vi "Mod_OFDM_Read_Configuration_From_File.vi"(0 "Configuration in":variant, 11 "error in":errorcluster) -> (4 "Configuration out":variant=variant("C"=variant(cluster{"Sub Carrier Selection":cluster{"Sub Carrier":bool, "Data Source":u16, "Modulator":u16}[], "OFDM Parameters":cluster{"# of Sub Carrier":i32, "Length Of Cylic Prefix":i32}} {"Sub Carrier Selection"=[{"Sub Carrier"=TRUE, "Data Source"=0, "Modulator"=0}, {"Sub Carrier"=TRUE, "Data Source"=0, "Modulator"=0}, {"Sub Carrier"=TRUE, "Data Source"=0, "Modulator"=0}, {"Sub Carrier"=TRUE, "Data Source"=0, "Modulator"=0}, {"Sub Carrier"=TRUE, "Data Source"=0, "Modulator"=0}, {"Sub Carrier"=TRUE, "Data Source"=0, "Modulator"=0}, {"Sub Carrier"=TRUE, "Data Source"=0, "Modulator"=0}, {"Sub Carrier"=TRUE, "Data Source"=0, "Modulator"=0}, {"Sub Carrier"=TRUE, "Data Source"=0, "Modulator"=0}, {"Sub Carrier"=TRUE, "Data Source"=0, "Modulator"=0}, {"Sub Carrier"=FALSE, "Data Source"=0, "Modulator"=0}, {"Sub Carrier"=FALSE, "Data Source"=0, "Modulator"=0}, {"Sub Carrier"=FALSE, "Data Source"=0, "Modulator"=0}, {"Sub Carrier"=FALSE, "Data Source"=0, "Modulator"=0}, {"Sub Carrier"=FALSE, "Data Source"=0, "Modulator"=0}, {"Sub Carrier"=FALSE, "Data Source"=0, "Modulator"=0}, {"Sub Carrier"=FALSE, "Data Source"=0, "Modulator"=0}, {"Sub Carrier"=FALSE, "Data Source"=0, "Modulator"=0}, {"Sub Carrier"=FALSE, "Data Source"=0, "Modulator"=0}, {"Sub Carrier"=FALSE, "Data Source"=0, "Modulator"=0}, {"Sub Carrier"=FALSE, "Data Source"=0, "Modulator"=0}, {"Sub Carrier"=FALSE, "Data Source"=0, "Modulator"=0}, {"Sub Carrier"=FALSE, "Data Source"=0, "Modulator"=0}, {"Sub Carrier"=FALSE, "Data Source"=0, "Modulator"=0}, {"Sub Carrier"=FALSE, "Data Source"=0, "Modulator"=0}, {"Sub Carrier"=FALSE, "Data Source"=0, "Modulator"=0}, {"Sub Carrier"=FALSE, "Data Source"=0, "Modulator"=0}, {"Sub Carrier"=FALSE, "Data Source"=0, "Modulator"=0}, {"Sub Carrier"=FALSE, "Data Source"=0, "Modulator"=0}, {"Sub Carrier"=FALSE, "Data Source"=0, "Modulator"=0}, {"Sub Carrier"=FALSE, "Data Source"=0, "Modulator"=0}, {"Sub Carrier"=TRUE, "Data Source"=0, "Modulator"=0}, {"Sub Carrier"=TRUE, "Data Source"=0, "Modulator"=0}, {"Sub Carrier"=TRUE, "Data Source"=0, "Modulator"=0}, {"Sub Carrier"=TRUE, "Data Source"=0, "Modulator"=0}, {"Sub Carrier"=TRUE, "Data Source"=0, "Modulator"=0}, {"Sub Carrier"=TRUE, "Data Source"=0, "Modulator"=0}, {"Sub Carrier"=TRUE, "Data Source"=0, "Modulator"=0}, {"Sub Carrier"=TRUE, "Data Source"=0, "Modulator"=0}, {"Sub Carrier"=TRUE, "Data Source"=0, "Modulator"=0}, {"Sub Carrier"=TRUE, "Data Source"=0, "Modulator"=0}, {"Sub Carrier"=TRUE, "Data Source"=0, "Modulator"=0}, {"Sub Carrier"=TRUE, "Data Source"=0, "Modulator"=0}, {"Sub Carrier"=TRUE, "Data Source"=0, "Modulator"=0}, {"Sub Carrier"=TRUE, "Data Source"=0, "Modulator"=0}, {"Sub Carrier"=TRUE, "Data Source"=0, "Modulator"=0}, {"Sub Carrier"=TRUE, "Data Source"=0, "Modulator"=0}, {"Sub Carrier"=TRUE, "Data Source"=0, "Modulator"=0}, {"Sub Carrier"=TRUE, "Data Source"=0, "Modulator"=0}, {"Sub Carrier"=TRUE, "Data Source"=0, "Modulator"=0}, {"Sub Carrier"=TRUE, "Data Source"=0, "Modulator"=0}, {"Sub Carrier"=TRUE, "Data Source"=0, "Modulator"=0}, {"Sub Carrier"=TRUE, "Data Source"=0, "Modulator"=0}, {"Sub Carrier"=TRUE, "Data Source"=0, "Modulator"=0}, {"Sub Carrier"=TRUE, "Data Source"=0, "Modulator"=0}, {"Sub Carrier"=TRUE, "Data Source"=0, "Modulator"=0}, {"Sub Carrier"=TRUE, "Data Source"=0, "Modulator"=0}, {"Sub Carrier"=TRUE, "Data Source"=0, "Modulator"=0}, {"Sub Carrier"=TRUE, "Data Source"=0, "Modulator"=0}, {"Sub Carrier"=TRUE, "Data Source"=0, "Modulator"=0}, {"Sub Carrier"=TRUE, "Data Source"=0, "Modulator"=0}, {"Sub Carrier"=TRUE, "Data Source"=0, "Modulator"=0}, {"Sub Carrier"=TRUE, "Data Source"=0, "Modulator"=0}, {"Sub Carrier"=TRUE, "Data Source"=0, "Modulator"=0}], "OFDM Parameters"={"# of Sub Carrier"=64, "Length Of Cylic Prefix"=16}}), "Data Source Pool "=variant(cluster{"mode (PN)":enum16{"PN", "pattern", "user"}, "PN sequence order (9)":i32, "base bit pattern (00001111)":enum16{"0", "1", "01", "0011", "00001111"}, "User base bit pattern":i8[]}[] [{"mode (PN)"=enum."PN", "PN sequence order (9)"=9, "base bit pattern (00001111)"=enum."00001111", "User base bit pattern"=[]}, {"mode (PN)"=enum."PN", "PN sequence order (9)"=9, "base bit pattern (00001111)"=enum."00001111", "User base bit pattern"=[]}, {"mode (PN)"=enum."PN", "PN sequence order (9)"=9, "base bit pattern (00001111)"=enum."00001111", "User base bit pattern"=[]}, {"mode (PN)"=enum."PN", "PN sequence order (9)"=9, "base bit pattern (00001111)"=enum."00001111", "User base bit pattern"=[]}, {"mode (PN)"=enum."PN", "PN sequence order (9)"=9, "base bit pattern (00001111)"=enum."00001111", "User base bit pattern"=[]}, {"mode (PN)"=enum."PN", "PN sequence order (9)"=9, "base bit pattern (00001111)"=enum."00001111", "User base bit pattern"=[]}]), "FRAME Table"=variant(string[][] [["C", "1"]]), "Modulator Source Pool "=variant(cluster{"M-QAM":enum16{"4", "16", "64", "256", "1024"}, "M-PSK":enum16{"2", "4", "8", "16", "32", "64", "128", "256"}, "Type of Modulation":enum16{"PSK", "QAM"}, "PSK":cluster{"differential PSK":enum16{"disable", "enable"}, "PSK type":u16}}[] [{"M-QAM"=enum."4", "M-PSK"=enum."4", "Type of Modulation"=enum."PSK", "PSK"={"differential PSK"=enum."disable", "PSK type"=0}}, {"M-QAM"=enum."4", "M-PSK"=enum."4", "Type of Modulation"=enum."PSK", "PSK"={"differential PSK"=enum."disable", "PSK type"=0}}, {"M-QAM"=enum."4", "M-PSK"=enum."4", "Type of Modulation"=enum."PSK", "PSK"={"differential PSK"=enum."disable", "PSK type"=0}}, {"M-QAM"=enum."4", "M-PSK"=enum."4", "Type of Modulation"=enum."PSK", "PSK"={"differential PSK"=enum."disable", "PSK type"=0}}, {"M-QAM"=enum."4", "M-PSK"=enum."4", "Type of Modulation"=enum."PSK", "PSK"={"differential PSK"=enum."disable", "PSK type"=0}}, {"M-QAM"=enum."4", "M-PSK"=enum."2", "Type of Modulation"=enum."PSK", "PSK"={"differential PSK"=enum."disable", "PSK type"=0}}]), "OFDM Frame"=variant(cluster{"Symbol Name":string, "# of Symbols":i32}[] [{"Symbol Name"="C", "# of Symbols"=1}]), "OFDM SYMBOL POOL"=variant(string[] ["C"]), "Pulse Shaping"=variant(cluster{"System Filter":cluster{"TX Filter":enum16{"none", "Raised Cosine", "Root Raised Cos"}, "Alpha":dbl, "filter length":i32}, "Modulation system parameters":cluster{"samples per symbol (16)":i32}, "symbol rate (Hz)":dbl} {"System Filter"={"TX Filter"=enum."Raised Cosine", "Alpha"=0.5, "filter length"=8}, "Modulation system parameters"={"samples per symbol (16)"=16}, "symbol rate (Hz)"=1.0}), "Sub Carrier Selection"=variant(cluster{"Sub Carrier Selection":cluster{"Sub Carrier":bool, "Data Source":u16, "Modulator":u16}[], "OFDM Parameters":cluster{"# of Sub Carrier":i32, "Length Of Cylic Prefix":i32}} {"Sub Carrier Selection"=[{"Sub Carrier"=TRUE, "Data Source"=0, "Modulator"=0}, {"Sub Carrier"=TRUE, "Data Source"=0, "Modulator"=0}, {"Sub Carrier"=TRUE, "Data Source"=0, "Modulator"=0}, {"Sub Carrier"=TRUE, "Data Source"=0, "Modulator"=0}, {"Sub Carrier"=TRUE, "Data Source"=0, "Modulator"=0}, {"Sub Carrier"=TRUE, "Data Source"=0, "Modulator"=0}, {"Sub Carrier"=TRUE, "Data Source"=0, "Modulator"=0}, {"Sub Carrier"=TRUE, "Data Source"=0, "Modulator"=0}, {"Sub Carrier"=TRUE, "Data Source"=0, "Modulator"=0}, {"Sub Carrier"=TRUE, "Data Source"=0, "Modulator"=0}, {"Sub Carrier"=TRUE, "Data Source"=0, "Modulator"=0}, {"Sub Carrier"=TRUE, "Data Source"=0, "Modulator"=0}, {"Sub Carrier"=TRUE, "Data Source"=0, "Modulator"=0}, {"Sub Carrier"=TRUE, "Data Source"=0, "Modulator"=0}, {"Sub Carrier"=TRUE, "Data Source"=0, "Modulator"=0}, {"Sub Carrier"=TRUE, "Data Source"=0, "Modulator"=0}, {"Sub Carrier"=TRUE, "Data Source"=0, "Modulator"=0}, {"Sub Carrier"=TRUE, "Data Source"=0, "Modulator"=0}, {"Sub Carrier"=TRUE, "Data Source"=0, "Modulator"=0}, {"Sub Carrier"=TRUE, "Data Source"=0, "Modulator"=0}, {"Sub Carrier"=TRUE, "Data Source"=0, "Modulator"=0}, {"Sub Carrier"=TRUE, "Data Source"=0, "Modulator"=0}, {"Sub Carrier"=TRUE, "Data Source"=0, "Modulator"=0}, {"Sub Carrier"=TRUE, "Data Source"=0, "Modulator"=0}, {"Sub Carrier"=TRUE, "Data Source"=0, "Modulator"=0}, {"Sub Carrier"=TRUE, "Data Source"=0, "Modulator"=0}, {"Sub Carrier"=TRUE, "Data Source"=0, "Modulator"=0}, {"Sub Carrier"=TRUE, "Data Source"=0, "Modulator"=0}, {"Sub Carrier"=TRUE, "Data Source"=0, "Modulator"=0}, {"Sub Carrier"=TRUE, "Data Source"=0, "Modulator"=0}, {"Sub Carrier"=TRUE, "Data Source"=0, "Modulator"=0}, {"Sub Carrier"=TRUE, "Data Source"=0, "Modulator"=0}, {"Sub Carrier"=TRUE, "Data Source"=0, "Modulator"=0}, {"Sub Carrier"=TRUE, "Data Source"=0, "Modulator"=0}, {"Sub Carrier"=TRUE, "Data Source"=0, "Modulator"=0}, {"Sub Carrier"=TRUE, "Data Source"=0, "Modulator"=0}, {"Sub Carrier"=TRUE, "Data Source"=0, "Modulator"=0}, {"Sub Carrier"=TRUE, "Data Source"=0, "Modulator"=0}, {"Sub Carrier"=TRUE, "Data Source"=0, "Modulator"=0}, {"Sub Carrier"=TRUE, "Data Source"=0, "Modulator"=0}, {"Sub Carrier"=TRUE, "Data Source"=0, "Modulator"=0}, {"Sub Carrier"=TRUE, "Data Source"=0, "Modulator"=0}, {"Sub Carrier"=TRUE, "Data Source"=0, "Modulator"=0}, {"Sub Carrier"=TRUE, "Data Source"=0, "Modulator"=0}, {"Sub Carrier"=TRUE, "Data Source"=0, "Modulator"=0}, {"Sub Carrier"=TRUE, "Data Source"=0, "Modulator"=0}, {"Sub Carrier"=TRUE, "Data Source"=0, "Modulator"=0}, {"Sub Carrier"=TRUE, "Data Source"=0, "Modulator"=0}, {"Sub Carrier"=TRUE, "Data Source"=0, "Modulator"=0}, {"Sub Carrier"=TRUE, "Data Source"=0, "Modulator"=0}, {"Sub Carrier"=TRUE, "Data Source"=0, "Modulator"=0}, {"Sub Carrier"=TRUE, "Data Source"=0, "Modulator"=0}, {"Sub Carrier"=TRUE, "Data Source"=0, "Modulator"=0}, {"Sub Carrier"=TRUE, "Data Source"=0, "Modulator"=0}, {"Sub Carrier"=TRUE, "Data Source"=0, "Modulator"=0}, {"Sub Carrier"=TRUE, "Data Source"=0, "Modulator"=0}, {"Sub Carrier"=TRUE, "Data Source"=0, "Modulator"=0}, {"Sub Carrier"=TRUE, "Data Source"=0, "Modulator"=0}, {"Sub Carrier"=TRUE, "Data Source"=0, "Modulator"=0}, {"Sub Carrier"=TRUE, "Data Source"=0, "Modulator"=0}, {"Sub Carrier"=TRUE, "Data Source"=0, "Modulator"=0}, {"Sub Carrier"=TRUE, "Data Source"=0, "Modulator"=0}, {"Sub Carrier"=TRUE, "Data Source"=0, "Modulator"=0}, {"Sub Carrier"=TRUE, "Data Source"=0, "Modulator"=0}, {"Sub Carrier"=TRUE, "Data Source"=0, "Modulator"=0}, {"Sub Carrier"=TRUE, "Data Source"=0, "Modulator"=0}, {"Sub Carrier"=TRUE, "Data Source"=0, "Modulator"=0}, {"Sub Carrier"=TRUE, "Data Source"=0, "Modulator"=0}, {"Sub Carrier"=TRUE, "Data Source"=0, "Modulator"=0}, {"Sub Carrier"=TRUE, "Data Source"=0, "Modulator"=0}, {"Sub Carrier"=TRUE, "Data Source"=0, "Modulator"=0}, {"Sub Carrier"=TRUE, "Data Source"=0, "Modulator"=0}, {"Sub Carrier"=TRUE, "Data Source"=0, "Modulator"=0}, {"Sub Carrier"=TRUE, "Data Source"=0, "Modulator"=0}, {"Sub Carrier"=TRUE, "Data Source"=0, "Modulator"=0}, {"Sub Carrier"=TRUE, "Data Source"=0, "Modulator"=0}, {"Sub Carrier"=TRUE, "Data Source"=0, "Modulator"=0}, {"Sub Carrier"=TRUE, "Data Source"=0, "Modulator"=0}, {"Sub Carrier"=TRUE, "Data Source"=0, "Modulator"=0}, {"Sub Carrier"=TRUE, "Data Source"=0, "Modulator"=0}, {"Sub Carrier"=TRUE, "Data Source"=0, "Modulator"=0}, {"Sub Carrier"=TRUE, "Data Source"=0, "Modulator"=0}, {"Sub Carrier"=TRUE, "Data Source"=0, "Modulator"=0}, {"Sub Carrier"=TRUE, "Data Source"=0, "Modulator"=0}, {"Sub Carrier"=TRUE, "Data Source"=0, "Modulator"=0}, {"Sub Carrier"=TRUE, "Data Source"=0, "Modulator"=0}, {"Sub Carrier"=TRUE, "Data Source"=0, "Modulator"=0}, {"Sub Carrier"=TRUE, "Data Source"=0, "Modulator"=0}, {"Sub Carrier"=TRUE, "Data Source"=0, "Modulator"=0}, {"Sub Carrier"=TRUE, "Data Source"=0, "Modulator"=0}, {"Sub Carrier"=TRUE, "Data Source"=0, "Modulator"=0}, {"Sub Carrier"=TRUE, "Data Source"=0, "Modulator"=0}, {"Sub Carrier"=TRUE, "Data Source"=0, "Modulator"=0}, {"Sub Carrier"=TRUE, "Data Source"=0, "Modulator"=0}, {"Sub Carrier"=TRUE, "Data Source"=0, "Modulator"=0}, {"Sub Carrier"=TRUE, "Data Source"=0, "Modulator"=0}, {"Sub Carrier"=TRUE, "Data Source"=0, "Modulator"=0}, {"Sub Carrier"=TRUE, "Data Source"=0, "Modulator"=0}, {"Sub Carrier"=TRUE, "Data Source"=0, "Modulator"=0}, {"Sub Carrier"=TRUE, "Data Source"=0, "Modulator"=0}, {"Sub Carrier"=TRUE, "Data Source"=0, "Modulator"=0}, {"Sub Carrier"=TRUE, "Data Source"=0, "Modulator"=0}, {"Sub Carrier"=TRUE, "Data Source"=0, "Modulator"=0}, {"Sub Carrier"=TRUE, "Data Source"=0, "Modulator"=0}, {"Sub Carrier"=TRUE, "Data Source"=0, "Modulator"=0}, {"Sub Carrier"=TRUE, "Data Source"=0, "Modulator"=0}, {"Sub Carrier"=TRUE, "Data Source"=0, "Modulator"=0}, {"Sub Carrier"=TRUE, "Data Source"=0, "Modulator"=0}, {"Sub Carrier"=TRUE, "Data Source"=0, "Modulator"=0}, {"Sub Carrier"=TRUE, "Data Source"=0, "Modulator"=0}, {"Sub Carrier"=TRUE, "Data Source"=0, "Modulator"=0}, {"Sub Carrier"=TRUE, "Data Source"=0, "Modulator"=0}, {"Sub Carrier"=TRUE, "Data Source"=0, "Modulator"=0}, {"Sub Carrier"=TRUE, "Data Source"=0, "Modulator"=0}, {"Sub Carrier"=TRUE, "Data Source"=0, "Modulator"=0}, {"Sub Carrier"=TRUE, "Data Source"=0, "Modulator"=0}, {"Sub Carrier"=TRUE, "Data Source"=0, "Modulator"=0}, {"Sub Carrier"=TRUE, "Data Source"=0, "Modulator"=0}, {"Sub Carrier"=TRUE, "Data Source"=0, "Modulator"=0}, {"Sub Carrier"=TRUE, "Data Source"=0, "Modulator"=0}, {"Sub Carrier"=TRUE, "Data Source"=0, "Modulator"=0}, {"Sub Carrier"=TRUE, "Data Source"=0, "Modulator"=0}, {"Sub Carrier"=TRUE, "Data Source"=0, "Modulator"=0}, {"Sub Carrier"=TRUE, "Data Source"=0, "Modulator"=0}, {"Sub Carrier"=TRUE, "Data Source"=0, "Modulator"=0}, {"Sub Carrier"=TRUE, "Data Source"=0, "Modulator"=0}, {"Sub Carrier"=TRUE, "Data Source"=0, "Modulator"=0}, {"Sub Carrier"=TRUE, "Data Source"=0, "Modulator"=0}], "OFDM Parameters"={"# of Sub Carrier"=64, "Length Of Cylic Prefix"=16}}), "Symbol Table"=variant(string[][] [["0", " ON", "0", "0"], ["1", " ON", "0", "0"], ["2", " ON", "0", "0"], ["3", " ON", "0", "0"], ["4", " ON", "0", "0"], ["5", " ON", "0", "0"], ["6", " ON", "0", "0"], ["7", " ON", "0", "0"], ["8", " ON", "0", "0"], ["9", " ON", "0", "0"], ["10", "OFF", "0", "0"], ["11", "OFF", "0", "0"], ["12", "OFF", "0", "0"], ["13", "OFF", "0", "0"], ["14", "OFF", "0", "0"], ["15", "OFF", "0", "0"], ["16", "OFF", "0", "0"], ["17", "OFF", "0", "0"], ["18", "OFF", "0", "0"], ["19", "OFF", "0", "0"], ["20", "OFF", "0", "0"], ["21", "OFF", "0", "0"], ["22", "OFF", "0", "0"], ["23", "OFF", "0", "0"], ["24", "OFF", "0", "0"], ["25", "OFF", "0", "0"], ["26", "OFF", "0", "0"], ["27", "OFF", "0", "0"], ["28", "OFF", "0", "0"], ["29", "OFF", "0", "0"], ["30", "OFF", "0", "0"], ["31", " ON", "0", "0"], ["32", " ON", "0", "0"], ["33", " ON", "0", "0"], ["34", " ON", "0", "0"], ["35", " ON", "0", "0"], ["36", " ON", "0", "0"], ["37", " ON", "0", "0"], ["38", " ON", "0", "0"], ["39", " ON", "0", "0"], ["40", " ON", "0", "0"], ["41", " ON", "0", "0"], ["42", " ON", "0", "0"], ["43", " ON", "0", "0"], ["44", " ON", "0", "0"], ["45", " ON", "0", "0"], ["46", " ON", "0", "0"], ["47", " ON", "0", "0"], ["48", " ON", "0", "0"], ["49", " ON", "0", "0"], ["50", " ON", "0", "0"], ["51", " ON", "0", "0"], ["52", " ON", "0", "0"], ["53", " ON", "0", "0"], ["54", " ON", "0", "0"], ["55", " ON", "0", "0"], ["56", " ON", "0", "0"], ["57", " ON", "0", "0"], ["58", " ON", "0", "0"], ["59", " ON", "0", "0"], ["60", " ON", "0", "0"], ["61", " ON", "0", "0"], ["62", " ON", "0", "0"], ["63", " ON", "0", "0"]])), 15 "error out":errorcluster)   [LabVIEW 2010]
doc: "Allows the user to load a pre-configured saved file. The VI loads all the settings upto the Pulse shaping parameters. \n\nNote: All the current configuration is lost if the VI is executed. The current settings are over written by the file which is read by the VI."
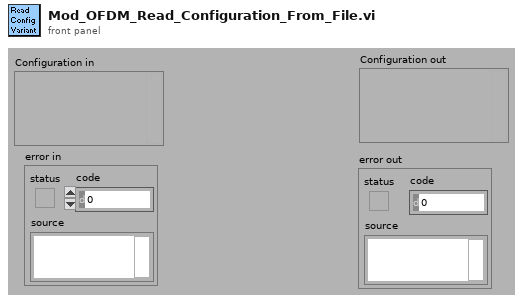
[diagram p1: front panel]
types:
  T1 = enum16{"open", "open or create", "create or replace", "create", "open (read only)"}
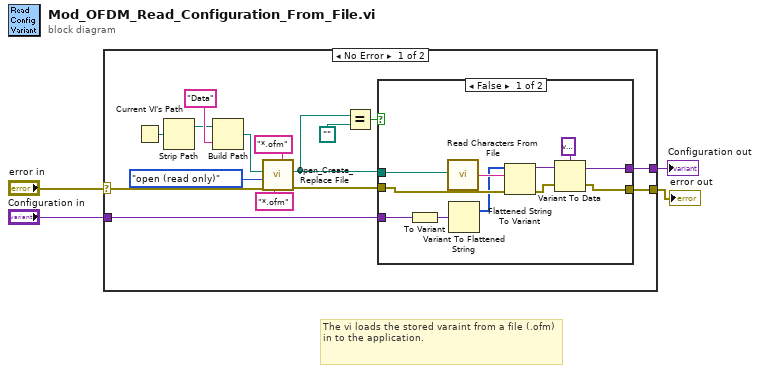
[diagram p0: block diagram]
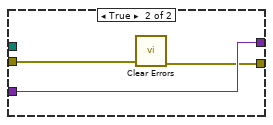
[diagram p2: hidden frame]
diagram:
  # "The vi loads the stored varaint from a file (.ofm) in to the application."
  n1 = case shown="No Error" "error in" {
    selector: "error in" -> [w7 w34]
    tunnel: [w14 w34] -> w4
    tunnel: [w13 _] -> w3
    tunnel: "Configuration in" -> [w12 _]
    frame No Error {
      n2 = Current VI's Path() -> (path=w9:path)
      n3 = Strip Path(path=w9) -> (stripped path=w10:path)  [unwired: 1 out]
      n4 = Build Path(base path=w10, name or relative path="Data") -> (appended path=w8:path)
      n5 = call <vilib>:"Open_Create_Replace File.vi"("pattern"="*.ofm", "default name"="*.ofm", "error in (no error)"=w7, "function (open:0)"=T1."open (read only)", "start path  (Not A Path)"=w8) -> ("error out"=w15:errorcluster, "new file path"=w6:path)  [unwired: 3 in, 2 out]
      n6 = Equal?(x=w6, y=path "") -> (x = y?=w16:bool)
      n7 = case shown="False" w16 {
        tunnel: w6 -> [w26 _]
        tunnel: w15 -> [w25 w32]
        tunnel: [w24 w31] -> w14
        tunnel: [w23 w33] -> w13
        tunnel: w12 -> [w22 w33]
        frame False {
          n8 = To Variant(anything=w22) -> (Variant=w21:variant)
          n9 = call <vilib>:"Read Characters From File.vi"("file path (dialog if empty)"=w26) -> ("character string"=w30:string)  [unwired: 5 in, 3 out]
          n10 = Variant To Flattened String(Variant=w21) -> (1:w20:i16[])  [unwired: 1 out]
          n11 = Flattened String To Variant(4:w25, 6:w30, 7:w20) -> (0:w29:errorcluster, 3:w27:variant)
          n12 = Variant To Data(error in=w29, Variant=w27, type=variant ("Variant")) -> (error out=w24:errorcluster, data=w23:variant)
        }
        frame True {
          n13 = call <vilib>:"Clear Errors.vi"("error in (no error)"=w32) -> ("error out"=w31:errorcluster)  [unwired: 6 in]
        }
      }
    }
    frame Error {
    }
  }
  "Configuration out" <- w3
  "error out" <- w4
